vi "array -- generate range -- V5.vi"(7 "action":T1, 8 "ω points":i32=100, 9 "ω from":dbl=1000.0, 10 "ω to":dbl=1000.0) -> (3 "ω out":dbl[](array[numeric])=[32012.991918577427, 32390.261658505893, 32466.39798177853, 32499.14340521798, 32517.39286113775, 32529.046092051318, 32537.14525712326, 32543.111142615544, 32547.696343954158, 32551.33675949651, 32554.302325209504, 32556.769142360055, 32558.856995237307, 32560.650202739795, 32562.209843476354, 32563.58125099723, 32564.7987833122, 32565.88895894197, 32566.872575330308, 32567.766175404246, 32568.583086316496, 32569.334166794306, 32570.02835688638, 32570.673085530187, 32571.274580490695, 32571.838104118455, 32572.36813539066, 32572.868514009202, 32573.342552524307, 32573.793126289274, 32574.222746575288, 32574.633618125405, 32575.027687968828, 32575.40668442971, 32575.772149741057, 32576.12546690325, 32576.467883345118, 32576.800529469096, 32577.124435064776, 32577.440543590797, 32577.749724325146, 32578.052781957467, 32578.35046682089, 32578.643482565894, 32578.932492128843, 32579.218126471686, 32579.500987779396, 32579.781656707495, 32580.06069600583, 32580.338656060805, 32580.616078519142, 32580.89350097748, 32581.171461032456, 32581.45050033079, 32581.73116925889, 32582.0140305666, 32582.29966469628, 32582.58867447239, 32582.88169000423, 32583.179375080817, 32583.48243271314, 32583.791613234323, 32584.10772197351, 32584.43162756919, 32584.764273480003, 32585.106690135035, 32585.460007297228, 32585.825472395412, 32586.204468856296, 32586.59853891288, 32587.009410462997, 32587.439030535847, 32587.889604513977, 32588.363642815923, 32588.86402143446, 32589.39405291983, 32589.957576334426, 32590.559071508098, 32591.203800151903, 32591.897990030815, 32592.64907072179, 32593.46598163404, 32594.359581707977, 32595.343197883154, 32596.433373726086, 32597.650906041054, 32599.022313348767, 32600.58195429849, 32602.375161800977, 32604.46301467823, 32606.929831615616, 32609.895397541775, 32613.535812870963, 32618.12101442274, 32624.086899701866, 32632.186064986967, 32643.839295900536, 32662.088751820305, 32694.834175046595, 32770.97049853239])   [LabVIEW 2021]
uses:
  array action.ctl
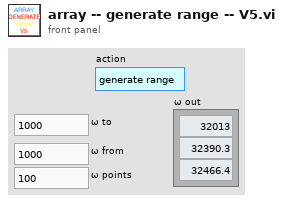
[diagram p1: front panel]
types:
  T1 = typedef "array action.ctl" = enum16{"generate range", "generate log range"}
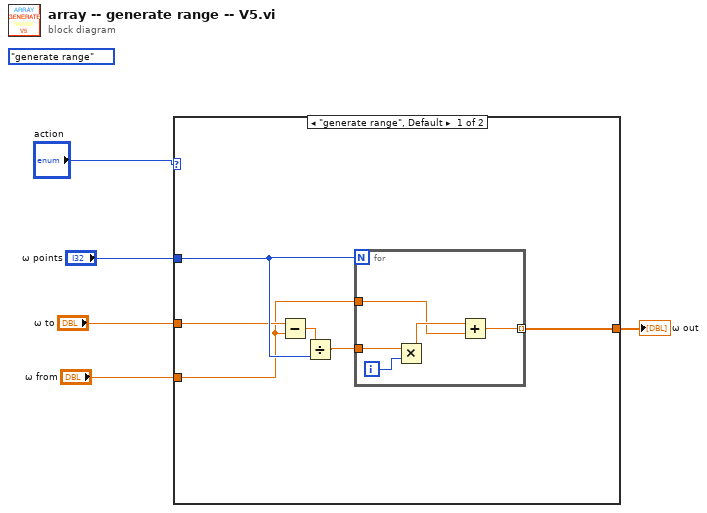
[diagram p0: block diagram]
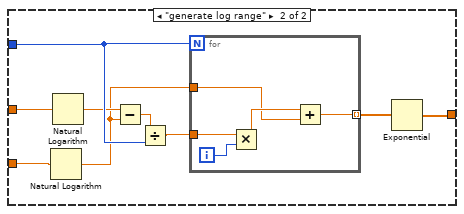
[diagram p2: hidden frame]
diagram:
  (unwired) array_action."generate range" ("action")
  n1 = case shown="\"generate range\", Default" "action" {
    tunnel: "ω points" -> [w11 w25]
    tunnel: [w9 w17] -> w4
    tunnel: "ω to" -> [w8 w22]
    tunnel: "ω from" -> [w6 w20]
    frame "generate range", Default {
      n2 = Subtract(x=w8, y=w6) -> (x-y=w7:dbl)
      n3 = Divide(x=w7, y=w11) -> (x/y=w10:dbl)
      n4 = for {
        N: w11 -> [_]
        tunnel: w10 -> [w15]
        tunnel: w6 -> [w13]
        tunnel: [w12] -> w9 mode=indexing
        i -> [w16]
        n5 = Multiply(x=w15, y=w16) -> (x*y=w14:dbl)
        n6 = Add(x=w14, y=w13) -> (x+y=w12:dbl)
      }
    }
    frame "generate log range" {
      n7 = Natural Logarithm(1:w20) -> (0:w19:dbl)
      n8 = Natural Logarithm(1:w22) -> (0:w21:dbl)
      n9 = Subtract(x=w21, y=w19) -> (x-y=w23:dbl)
      n10 = Divide(x=w23, y=w25) -> (x/y=w24:dbl)
      n11 = for {
        N: w25 -> [_]
        tunnel: w24 -> [w29]
        tunnel: w19 -> [w27]
        tunnel: [w26] -> w18 mode=indexing
        i -> [w30]
        n12 = Multiply(x=w29, y=w30) -> (x*y=w28:dbl)
        n13 = Add(x=w28, y=w27) -> (x+y=w26:dbl)
      }
      n14 = Exponential(1:w18) -> (0:w17:dbl[])
    }
  }
  "ω out" <- w4
